vi "Set Cal Expires.vi"(8 "error in (no error)":errorcluster, 10 "Cal Expires":timestamp, 11 "Device in":refnum<class "Device.lvclass">) -> (0 "error out":errorcluster, 3 "Device out":refnum<class "Device.lvclass">)   [LabVIEW 2020, in "HAL.lvlib" / "Device.lvclass"]
uses:
  Device.lvclass
  Device.lvclass/Device.ctl
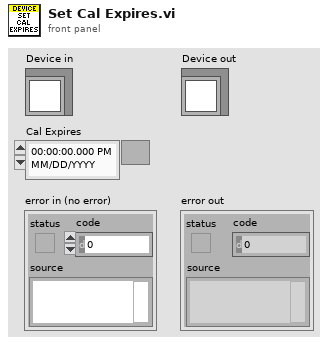
[diagram p1: front panel]
types:
  T1 = typedef "HAL.lvlib/Device.lvclass/Ref Data.ctl" = cluster{"Config Keys":string[], "Config Values":string[], "Cal Expires":timestamp, "Name":string, "Comment":string, "State":T2, "Error":errorcluster}
  T2 = typedef "HAL.lvlib/Device.lvclass/Device State.ctl" = enum16{"Uninitialized", "Initialized", "Running", "Error"}
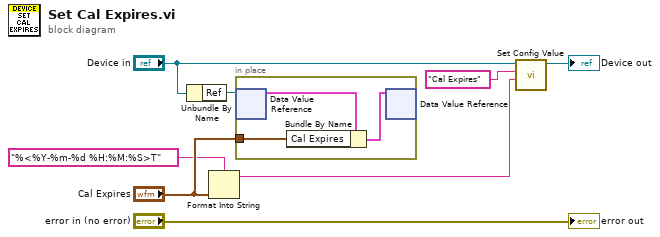
[diagram p0: block diagram]
diagram:
  n1 = Unbundle By Name("Device in") -> ("Ref"=w7:refnum<data-value>)
  n2 = Format Into String(format string="%<%Y-%m-%d %H:%M:%S>T", "Cal Expires") -> (resulting string=w1:string)  [unwired: 2 in, 1 out]
  n3 = in-place {
    in-place-border: "Cal Expires" -> [w9]
    n4 = in-place-dvr #1(w7) -> (w11:T1)  [unwired: 1 out]
    n5 = Bundle By Name(cluster=w11, "Cal Expires"=w9) -> (w10:T1)
    n6 = in-place-dvr #1(w10) -> ()  [unwired: 2 out]
  }
  n7 = call "Set Config Value.vi"("Value"=w1, "Config Key"="Cal Expires", "Device in"="Device in") -> ("Device out"=→"Device out":refnum<class "Device.lvclass">)  [unwired: 7 in, 1 out]
  "error out" <- "error in (no error)"
